vi "AO Write.vi"(7 "AO line":T1=5100 items=["ModB/AO0"=5100, "ModB/AO1"=5101, "ModB/AO2"=5102, "ModB/AO3"=5103], 8 "error in (no error)":errorcluster, 10 "data":dbl, 11 "direct IO in":refnum<class "NI_Robotics_Starter Kit Direct IO_FPGA.lvclass">) -> (0 "error out":errorcluster, 3 "direct IO out":refnum<class "NI_Robotics_Starter Kit Direct IO_FPGA.lvclass">)   [LabVIEW 2017, in "NI_Robotics_Starter Kit Direct IO_FPGA.lvclass"]
uses:
  <vilib>/robotics/Starter Kit/FPGA Direct IO/NI_Robotics_Starter Kit Direct IO_FPGA.lvclass
  <vilib>/robotics/Starter Kit/Direct IO/AO Lines.ctl
  <vilib>/robotics/Starter Kit/FPGA Direct IO/NI_Robotics_Starter Kit Direct IO_FPGA.lvclass/NI_Robotics_Starter Kit Direct IO_FPGA.ctl
  <vilib>/rvi/errors/niLvFpgaAdjustHostInterfaceError.vi
  <vilib>/Utility/error.llb/Error Cluster From Error Code.vi
  <vilib>/robotics/Starter Kit/FPGA Direct IO/Direct IO FPGA Ref.ctl
  <vilib>/rvi/interface/nirviReadWriteControl/nirviReadWriteControl.xnode
  NiFpgaLv.dll
  <vilib>/rvi/interface/Simulation/niFpgaSimulationCallBeginRW.vi
  <vilib>/robotics/Starter Kit/Direct IO/NI_Robotics_Starter Kit Direct IO.lvclass
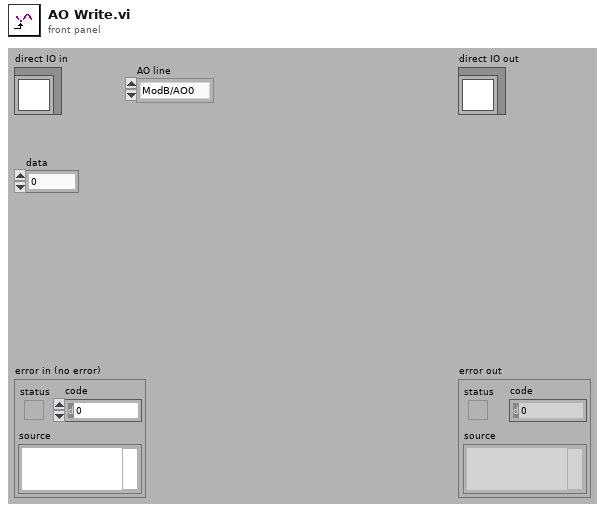
[diagram p1: front panel]
types:
  T1 = typedef "NI_Robotics_Starter Kit Direct IO.lvclass/AO Lines.ctl" = u16
  T2 = typedef "NI_Robotics_Starter Kit Direct IO_FPGA.lvclass/Direct IO FPGA Ref.ctl" = refnum<k20>
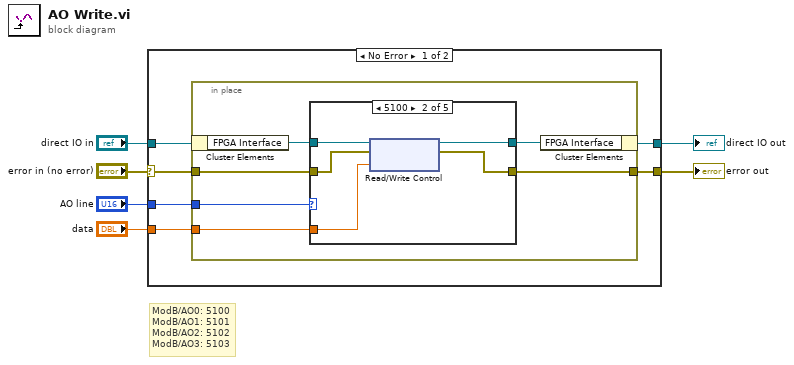
[diagram p0: block diagram]
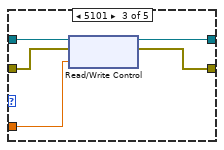
[diagram p3: hidden frame]
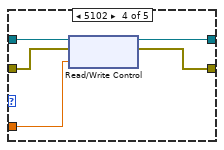
[diagram p4: hidden frame]
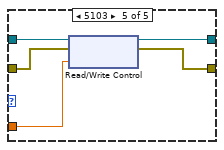
[diagram p5: hidden frame]
diagram:
  # "ModB/AO0: 5100\nModB/AO1: 5101\nModB/AO2: 5102\nModB/AO3: 5103"
  n1 = case shown="No Error" "error in (no error)" {
    selector: "error in (no error)" -> [w10 w42]
    tunnel: [w9 w42] -> w2
    tunnel: "direct IO in" -> [w12 w41]
    tunnel: [w8 w41] -> w3
    tunnel: "AO line" -> [w11 _]
    tunnel: "data" -> [w7 _]
    frame No Error {
      n2 = in-place {
        in-place-border: w11 -> [w18]
        in-place-border: w10 -> [w16]
        in-place-border: [w14] -> w9
        in-place-border: w7 -> [w13]
        n3 = in-place-cluster #1(w12) -> ("FPGA Interface"=w17:T2)
        n4 = case shown="5100" w18 {
          tunnel: w17 -> [w20 w25 w30 w35 w40]
          tunnel: w16 -> [w19 w24 w29 w34 w39]
          tunnel: [w20 w23 w28 w33 w38] -> w15
          tunnel: [w19 w22 w27 w32 w37] -> w14
          tunnel: w13 -> [_ w21 w26 w31 w36]
          frame Default {
          }
          frame 5100 {
            n5 = xnode "Read/Write Control"("FPGA VI Reference In"=w25, "error in"=w24, "ModB/AO0"=w21) -> ("FPGA VI Reference Out"=w23:T2, "error out"=w22:errorcluster)
          }
          frame 5101 {
            n6 = xnode "Read/Write Control"("FPGA VI Reference In"=w30, "error in"=w29, "ModB/AO1"=w26) -> ("FPGA VI Reference Out"=w28:T2, "error out"=w27:errorcluster)
          }
          frame 5102 {
            n7 = xnode "Read/Write Control"("FPGA VI Reference In"=w35, "error in"=w34, "ModB/AO2"=w31) -> ("FPGA VI Reference Out"=w33:T2, "error out"=w32:errorcluster)
          }
          frame 5103 {
            n8 = xnode "Read/Write Control"("FPGA VI Reference In"=w40, "error in"=w39, "ModB/AO3"=w36) -> ("FPGA VI Reference Out"=w38:T2, "error out"=w37:errorcluster)
          }
        }
        n9 = in-place-cluster #1("FPGA Interface"=w15) -> (w8:refnum<class "NI_Robotics_Starter Kit Direct IO_FPGA.lvclass">)
      }
    }
    frame Error {
    }
  }
  "error out" <- w2
  "direct IO out" <- w3
